vi "Warnings.vi"() -> (3 "Project name":string, 4 "Invalid project path":string, 6 "Incompatible project version":string, 8 "Invalid measurement path":string, 10 "Incompatible measurement version":string, 13 "Permission error":string, 14 "Invalid folder/file names":string, 15 "Drive selection":string)   [LabVIEW 2021, in "Migrator.lvlib"]
uses:
  Migrator.lvlib
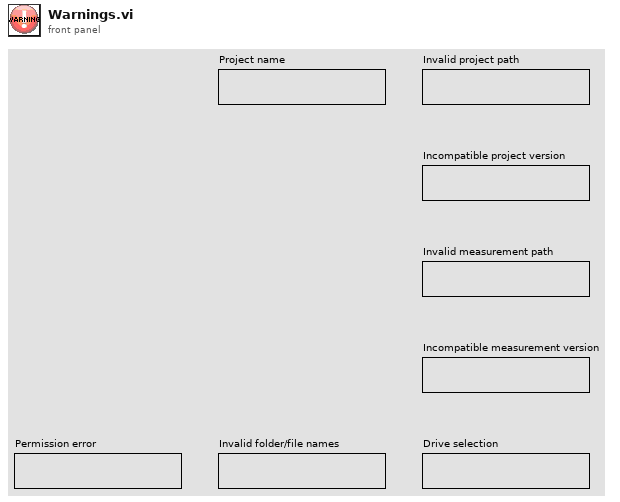
[diagram p1: front panel]
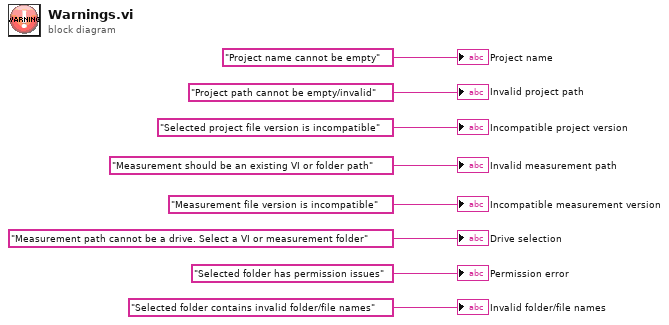
[diagram p0: block diagram]
diagram:
  "Invalid project path" <- "Project path cannot be empty/invalid" ("Invalid project path")
  "Incompatible project version" <- "Selected project file version is incompatible" ("Invalid project path")
  "Invalid measurement path" <- "Measurement should be an existing VI or folder path" ("Invalid project path")
  "Incompatible measurement version" <- "Measurement file version is incompatible" ("Invalid project path")
  "Drive selection" <- "Measurement path cannot be a drive. Select a VI or measurement folder" ("Invalid project path")
  "Project name" <- "Project name cannot be empty" ("Project name")
  "Permission error" <- "Selected folder has permission issues" ("Invalid project path")
  "Invalid folder/file names" <- "Selected folder contains invalid folder/file names" ("Invalid project path")
